vi "Obtain Hwnd-LV Dev.vi"(0 "LV DEV in":refnum<class "LV DEV.lvclass">, 11 "error in (no error)":errorcluster) -> (4 "LV DEV out":refnum<class "LV DEV.lvclass">, 15 "error out":errorcluster)   [LabVIEW 2016, in "LV DEV.lvclass"]
uses:
  LV DEV.lvclass
  D:/MDI Project/source code/Document/Child Classes/LV Doc/LV Doc.lvclass
  D:/MDI Project/source code/Document/Document.lvclass
  LV Doc.lvclass/LV Doc.ctl
  Document.lvclass/Document.ctl
  Document.lvclass
  LV Doc.lvclass
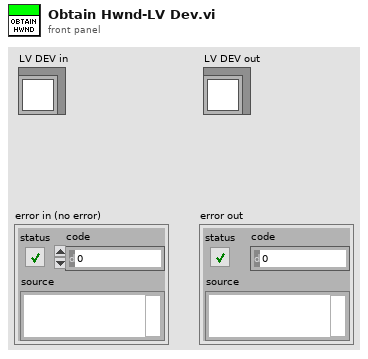
[diagram p1: front panel]
types:
  T1 = enum32{"Invalid", "Standard", "Closed", "Hidden", "Minimized", "Maximized"}
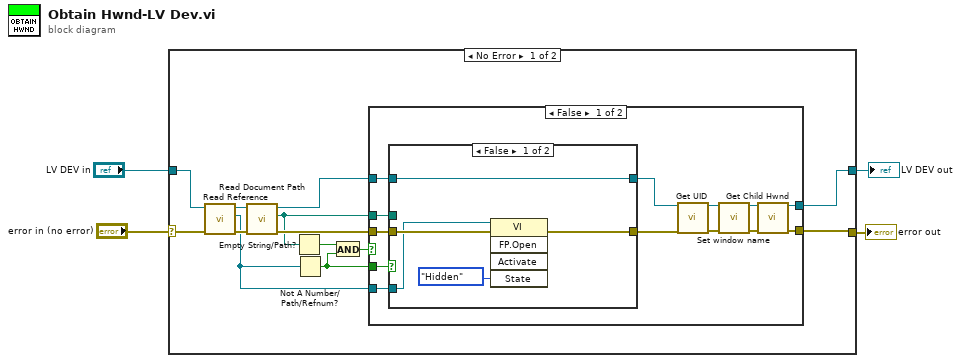
[diagram p0: block diagram]
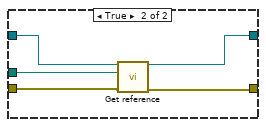
[diagram p2: hidden frame]
diagram:
  n1 = case shown="No Error" "error in (no error)" {
    selector: "error in (no error)" -> [w12 w43]
    tunnel: [w9 w43] -> w4
    tunnel: [w10 w44] -> w3
    tunnel: "LV DEV in" -> [w11 w44]
    frame No Error {
      n2 = call "Read Reference.vi"("error in (no error)"=w12, "LV Doc in"=w11) -> ("error out"=w15:errorcluster, "Reference"=w13:refnum<vi>, "LV Doc out"=w14:refnum<class "LV DEV.lvclass">)  [unwired: 7 in]
      n3 = call "Read Document Path.vi"("error in (no error)"=w15, "Document in"=w14) -> ("error out"=w16:errorcluster, "Document Path"=w8:path, "Document out"=w17:refnum<class "LV DEV.lvclass">)  [unwired: 7 in]
      n4 = Empty String/Path?(string/path=w8) -> (empty?=w7:bool)
      n5 = Not A Number/Path/Refnum?(number/path/refnum=w13) -> (NaN/Path/Refnum?=w6:bool)
      n6 = And(x=w7, y=w6) -> (x .and. y?=w5:bool)
      n7 = case shown="False" w5 {
        tunnel: w17 -> [w30 w42]
        tunnel: w16 -> [w29 w41]
        tunnel: w8 -> [w28 _]
        tunnel: w13 -> [w27 _]
        tunnel: [w26 w42] -> w10
        tunnel: [w25 w41] -> w9
        tunnel: w6 -> [w18 _]
        frame False {
          n8 = case shown="False" w18 {
            tunnel: [w32 w39] -> w20
            tunnel: w29 -> [w33 w40]
            tunnel: w28 -> [_ w38]
            tunnel: w27 -> [w31 _]
            tunnel: w30 -> [w35 w37]
            tunnel: [w35 w36] -> w19
            frame False {
              n9 = invoke class="VI" method="FP.Open"(reference=w31, error in=w33, "State"=T1."Hidden") -> (error out=w32:errorcluster)  [unwired: 2 in, 4 out]
            }
            frame True {
              n10 = call "Get reference.vi"("LV DEV.lvclass"=w37, "Vi Path"=w38, "Error in"=w40) -> ("LV DEV.lvclass"=w36:refnum<class "LV DEV.lvclass">, "Error Out"=w39:errorcluster)  [unwired: 11 in]
            }
          }
          n11 = call "Get UID.vi"("LV Doc.lvclass"=w19, "error in (no error)"=w20) -> ("LV Doc.lvclass"=w22:refnum<class "LV DEV.lvclass">, "error out"=w23:errorcluster)  [unwired: 12 in]
          n12 = call "Set window name.vi"("LV Doc.lvclass"=w22, "error in (no error)"=w23) -> ("LV Doc.lvclass"=w21:refnum<class "LV DEV.lvclass">, "error out"=w24:errorcluster)  [unwired: 12 in]
          n13 = call "Get Child Hwnd.vi"("LV Doc.lvclass"=w21, "Error in"=w24) -> ("LV Doc.lvclass"=w26:refnum<class "LV DEV.lvclass">, "Error Out"=w25:errorcluster)  [unwired: 12 in]
        }
        frame True {
        }
      }
    }
    frame Error {
    }
  }
  "error out" <- w4
  "LV DEV out" <- w3
